vi "Camera Tracking.vi"(9 "Was Tracking":bool, 11 "Shooter Controls":T1) -> (0 "Aligned":bool, 1 "Drive Y":dbl, 2 "Drive X":dbl format="%.2f", 3 "Shooter Controls Out":T1, 4 "Target Angle":dbl)   [LabVIEW 2011]
uses:
  Robot Global Data.vi
  <vilib>/addons/control/pid/NI_PID_pid.lvlib
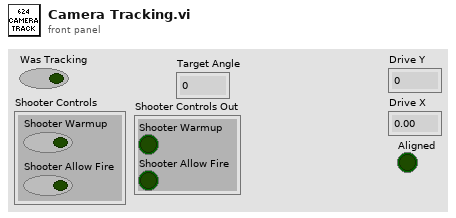
[diagram p1: front panel]
types:
  T1 = cluster{"Shooter Warmup":bool, "Shooter Allow Fire":bool}
  T2 = typedef "UDP Dashboard Packet TypeDef.ctl" = cluster{"Distance":dbl, "Shooter Control":cluster{"Manual Enabled":bool, "Manual Distance":dbl, "Power Constant":dbl, "RPM Constant":dbl, "Layup Distance":dbl, "RPM Range":cluster{"Max Percentage":dbl, "Min Percentage":dbl}, "Dt In":dbl}, "Tracking Setpoint":dbl, "Shooter PID gains":cluster{"proportional gain (Kc)":dbl, "integral time (Ti, min)":dbl, "derivative time (Td, min)":dbl}, "Tracking PID gains":cluster{"proportional gain (Kc)":dbl, "integral time (Ti, min)":dbl, "derivative time (Td, min)":dbl}, "Shooter PID gains 2":cluster{"proportional gain (Kc)":dbl, "integral time (Ti, min)":dbl, "derivative time (Td, min)":dbl}, "Tracking Tolerance":dbl, "Tracking Limit":dbl, "Autonomous Ball Collection / Shoot Period":dbl}
  T3 = cluster{"proportional gain (Kc)":dbl, "integral time (Ti, min)":dbl, "derivative time (Td, min)":dbl}
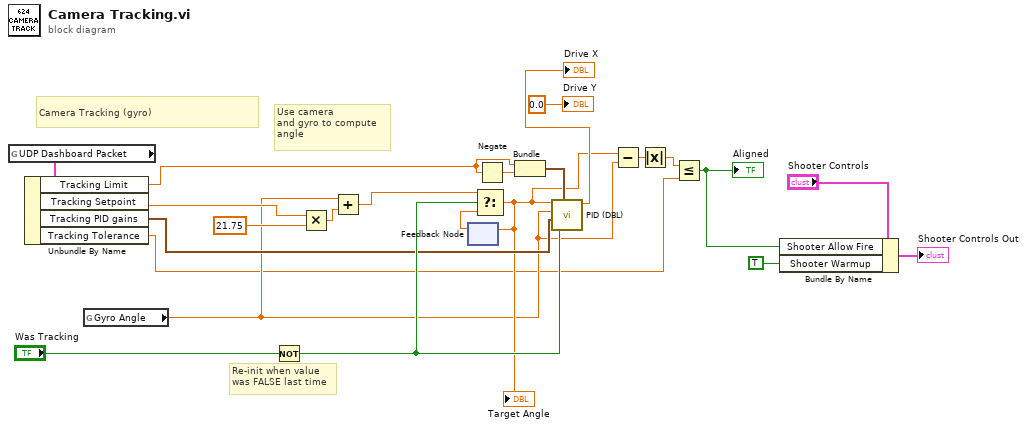
[diagram p0: block diagram]
diagram:
  # "Camera Tracking (gyro)"
  # "Re-init when value\nwas FALSE last time"
  # "Use camera\nand gyro to compute\nangle"
  n1 = global read "Robot Global Data.vi" "UDP Dashboard Packet"() -> (w17:T2)
  n2 = Unbundle By Name(w17) -> ("Tracking Limit"=w1:dbl, "Tracking Setpoint"=w16:dbl, "Tracking PID gains"=w13:T3, "Tracking Tolerance"=w8:dbl)
  n3 = global read "Robot Global Data.vi" "Gyro Angle"() -> (w9:dbl)
  n4 = Not(x="Was Tracking") -> (.not. x?=w14:bool)
  n5 = Multiply(x=w16, y=sgl 21.75 ("deg full screen 2")) -> (x*y=w20:dbl)
  n6 = Add(x=w9, y=w20) -> (x+y=w18:dbl)
  n7 = feedback #1() -> (w19:dbl)  [unwired: 1 out]
  n8 = Select(t=w18, s=w14, f=w19) -> (s? t:f=w10:dbl)
  "Target Angle" <- w10
  n9 = feedback-in #1(w10) -> ()
  n10 = Negate(x=w1) -> (-x=w23:dbl)
  n11 = Bundle("Tracking Limit"=w1, w23) -> (w22:cluster{"Tracking Limit":dbl, dbl})  [unwired: 1 out]
  n12 = call <vilib>:"PID (DBL).vi"("reinitialize? (F)"=w14, "output range"=w22, "PID gains"=w13, "process variable"=w9, "setpoint"=w10) -> ("output"=→"Drive X":dbl)  [unwired: 1 in, 5 out]
  n13 = Subtract(x=w10, y=w9) -> (x-y=w11:dbl)
  n14 = Absolute Value(x=w11) -> (abs(x)=w12:dbl)
  n15 = Less Or Equal?(x=w12, y=w8) -> (x <= y?=w2:bool)
  "Aligned" <- w2
  n16 = Bundle By Name(cluster="Shooter Controls", "Shooter Allow Fire"=w2, "Shooter Warmup"=TRUE ("Button 3")) -> (→"Shooter Controls Out":T1)
  "Drive Y" <- 0.0 ("axis 2 (y)")
